vi "Test Write.vi"() -> ()   [LabVIEW 2016, in "Control Experiment.lvclass"]
uses:
  Control Experiment.lvclass
  Control Experiment.lvclass/Control Experiment.ctl
panel:
  in  "stop":bool
  in  "Experiment.Device":string
  in  "Experiment.Device Path":path
  in  "Experiment Folder":string="6H_IVcurves"
  in  "Experiment Comments":string="SA03036H\nsweep Vsg:-150mV to 600mV, 1mV steps\nB: 7T to -7T\nVbg = -3.9V\nT: 50mK\n\nlockin\n\nI+/-: 2/3 3mV ac+ 250uV dc bias, 0.4 Hz\nV1+/-: 8/4\nV2+/- 6/28\nV3+/V3-: 27/8\nVsg: 1\nVbg :26\n\ntc 300ms order 2"
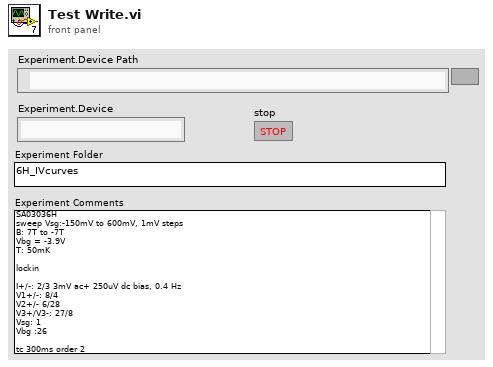
[diagram p1: front panel]
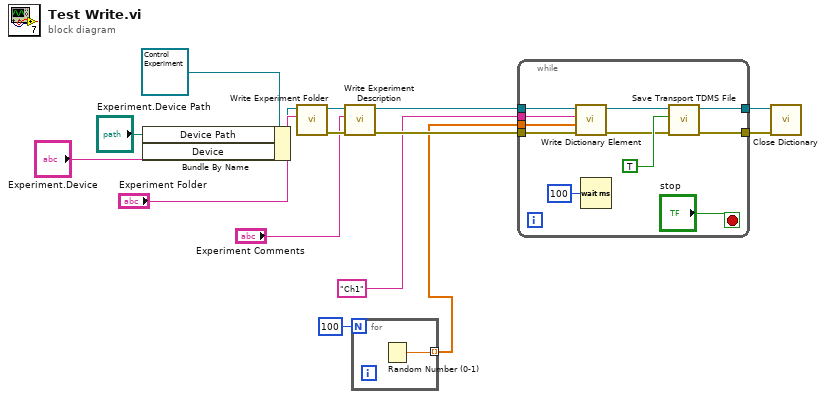
[diagram p0: block diagram]
diagram:
  n1 = Bundle By Name(cluster=refnum<class "Control Experiment.lvclass"> refnum ("Control Experiment in"), "Device Path"="Experiment.Device Path", "Device"="Experiment.Device") -> (w5:refnum<class "Control Experiment.lvclass">)
  n2 = call "Write Experiment Folder.vi"("Experiment Folder"="Experiment Folder", "Control Experiment in"=w5) -> ("error out"=w14:errorcluster, "Control Experiment out"=w15:refnum<class "Control Experiment.lvclass">)  [unwired: 8 in]
  n3 = call "Write Experiment Description.vi"("error in (no error)"=w14, "Experiment Description"="Experiment Comments", "Control Experiment in"=w15) -> ("error out"=w12:errorcluster, "Control Experiment out"=w11:refnum<class "Control Experiment.lvclass">)  [unwired: 7 in]
  n4 = for {
    N: 100 -> [_]
    tunnel: [w16] -> w7 mode=indexing
    n5 = Random Number (0-1)() -> (number: 0 to 1=w16:dbl)
  }
  n6 = while {
    tunnel: w12 -> [w24]
    tunnel: w11 -> [w23]
    tunnel: "Ch1" ("key") -> [w22]
    tunnel: w7 -> [w21]
    tunnel: [w19] -> w2
    tunnel: [w18] -> w1
    stop <- "stop" stop-if-true
    n7 = call "Write Dictionary Element.vi"("error in (no error)"=w24, "value"=w21, "key"=w22, "Control Experiment in"=w23) -> ("error out"=w25:errorcluster, "Control Experiment out"=w26:refnum<class "Control Experiment.lvclass">)  [unwired: 6 in]
    n8 = Wait (ms)(milliseconds to wait=u32 100) -> ()  [unwired: 1 out]
    n9 = call "Save Transport TDMS File.vi"("error in (no error)"=w25, "append?"=TRUE, "Control Experiment in"=w26) -> ("error out"=w19:errorcluster, "Control Experiment out"=w18:refnum<class "Control Experiment.lvclass">)  [unwired: 7 in]
  }
  n10 = call "Close Dictionary.vi"("error in (no error)"=w2, "Control Experiment in"=w1) -> ()  [unwired: 8 in, 2 out]
